vi "Configure Flow Rate Setpoint.vi"(8 "error in (no error)":errorcluster, 10 "flow rate setpoint, %":dbl, 11 "RRG in":refnum<class "PL Eltochpribor RRG.lvclass">) -> (0 "error out":errorcluster, 3 "RRG out":refnum<class "PL Eltochpribor RRG.lvclass">)   [LabVIEW 2015, in "PL Eltochpribor RRG.lvclass"]
doc: "Configures flow rate setpoint as a percentage of full scale calibrated flow rate."
uses:
  PL Eltochpribor RRG.lvclass
  <vilib>/plasmapper/PL Modbus Client/PL Modbus Client.lvclass
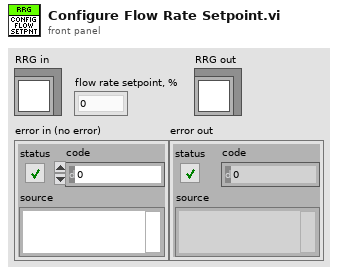
[diagram p1: front panel]
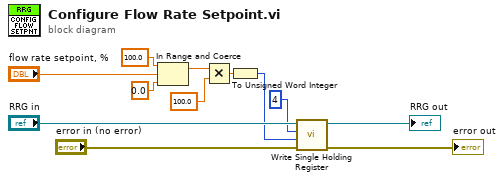
[diagram p0: block diagram]
diagram:
  n1 = In Range and Coerce(upper limit=100.0, x="flow rate setpoint, %", lower limit=0.0) -> (coerced(x)=w4:dbl)  [unwired: 1 out]
  n2 = Multiply(x=w4, y=100.0 ("upper limit")) -> (x*y=w2:dbl)
  n3 = To Unsigned Word Integer(number=w2) -> (unsigned 16bit integer=w1:u16)
  n4 = call <vilib>:"Write Single Holding Register.vi"("error in (no error)"="error in (no error)", "value"=w1, "address"=u16 4, "MODBUS in"="RRG in") -> ("error out"=→"error out":errorcluster, "MODBUS out"=→"RRG out":refnum<class "PL Eltochpribor RRG.lvclass">)  [unwired: 6 in]
